vi "Programas.vi"(8 "error in (no error)":errorcluster) -> (0 "error out":errorcluster, 3 "Message":string)   [LabVIEW 2014]
uses:
  controls/Programas/UI Entrenamiento.ctl
  controls/Programas/UI Metabolico.ctl
  controls/Programas/UI Activacion.ctl
  controls/Programas/UI Avatar.ctl
panel:
  out "date/time string":string
  in  "Help":bool
  in  "Reset":bool
  in  "Back":bool
  in  "Avatar":T1 caption="Date Time"
  in  "Activacion":T2
  in  "Metabolico":T3
  in  "Entrenamiento":T4
  # "Elija un Programa"
  # "Presentación"
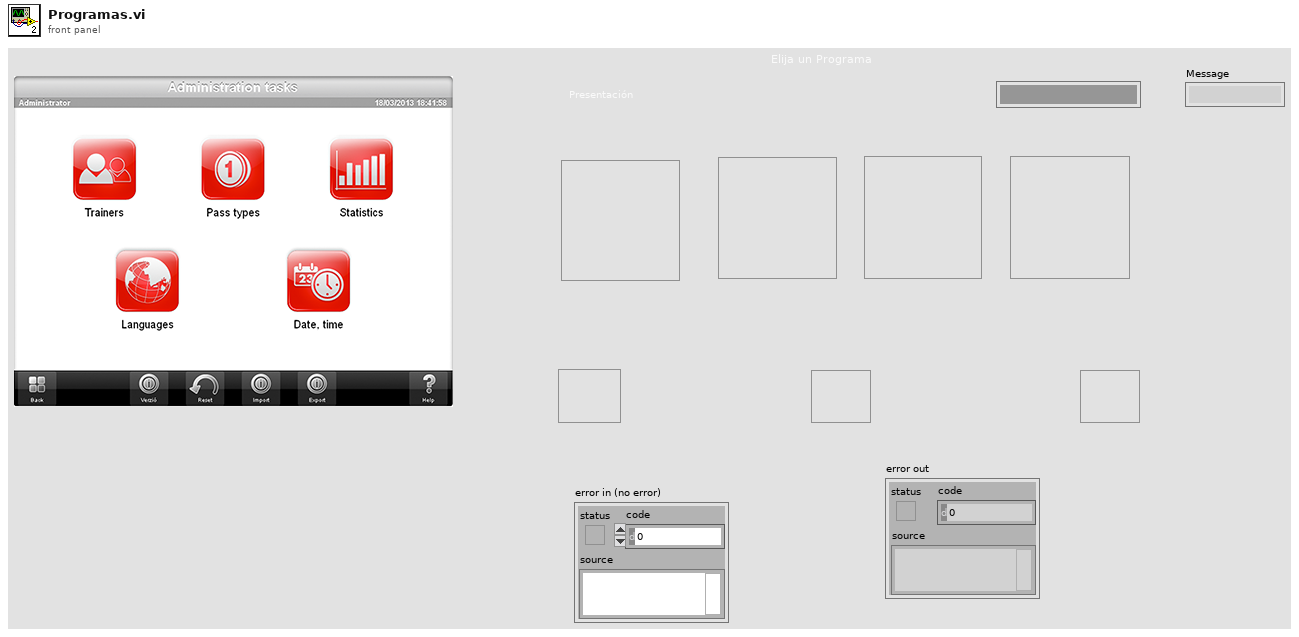
[diagram p1: front panel]
types:
  T1 = typedef "UI Avatar.ctl" = bool
  T2 = typedef "UI Activacion.ctl" = bool
  T3 = typedef "UI Metabolico.ctl" = bool
  T4 = typedef "UI Entrenamiento.ctl" = bool
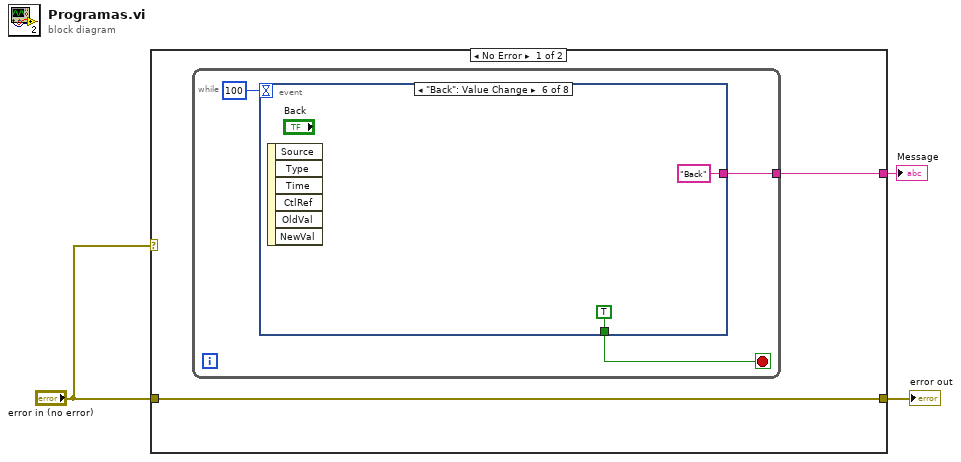
[diagram p0: block diagram]
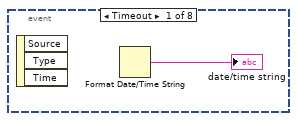
[diagram p2: hidden frame]
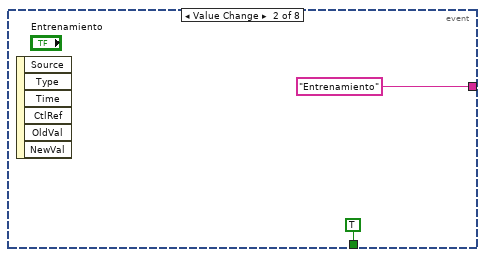
[diagram p3: hidden frame]
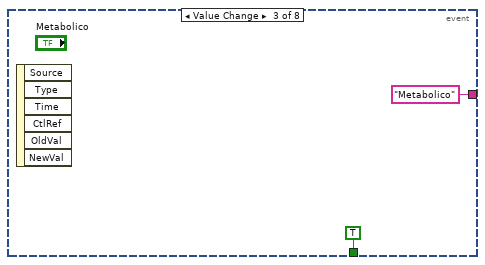
[diagram p4: hidden frame]
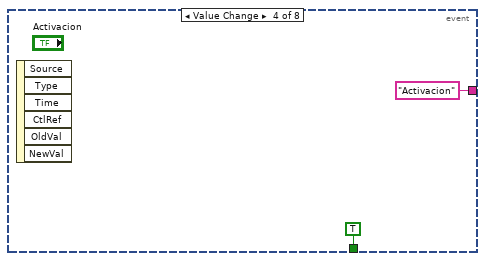
[diagram p5: hidden frame]
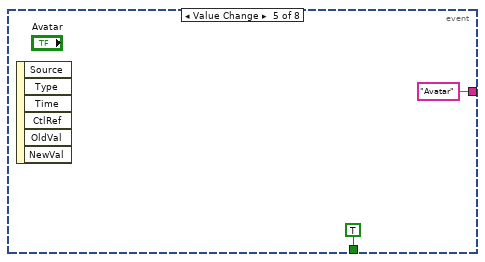
[diagram p6: hidden frame]
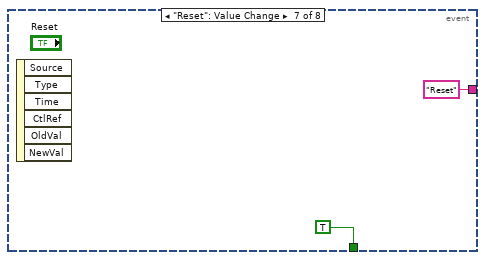
[diagram p7: hidden frame]
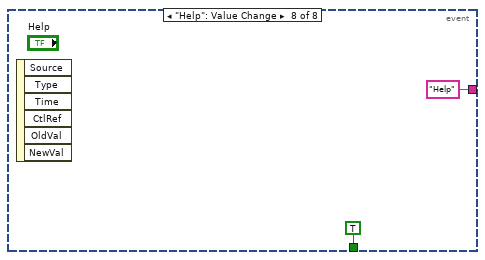
[diagram p8: hidden frame]
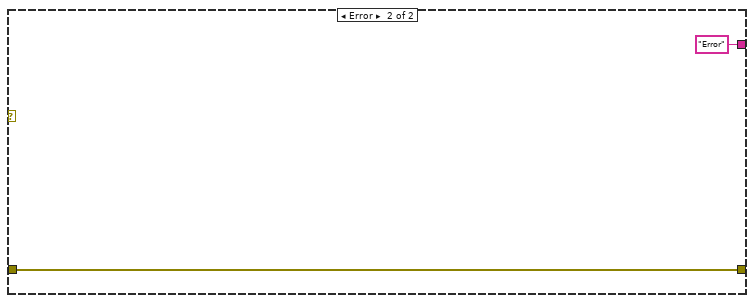
[diagram p9: hidden frame]
diagram:
  n1 = case shown="No Error" "error in (no error)" {
    tunnel: "error in (no error)" -> [w5 w25]
    tunnel: [w5 w25] -> w2
    tunnel: [w4 "Error" ("Message")] -> w1
    frame No Error {
      n2 = while {
        tunnel: [w6] -> w4
        stop <- w8 stop-if-true
        n3 = event shown="[5] \"Back\": Value Change" {
          selector: _ -> [_ _ _ _ _ _ _ _]
          dyn-events: _ -> [_ _ _ _ _ _ _ _]
          timeout: 100 -> [_ _ _ _ _ _ _ _]
          tunnel: [_ TRUE TRUE TRUE TRUE TRUE TRUE TRUE] -> w8
          tunnel: [_ "Entrenamiento" ("Message") "Metabolico" ("Message") "Activacion" ("Message") "Avatar" ("Message") "Back" ("Message") "Reset" ("Message") "Help" ("Message")] -> w6
          event Timeout {
            n4 = event-data() -> ()  [unwired: 1 in, 3 out]
            n5 = Format Date/Time String() -> (date/time string=→"date/time string":string)  [unwired: 3 in]
          }
          event Value Change {
            n6 = event-data() -> ()  [unwired: 1 in, 6 out]
          }
          event Value Change {
            n7 = event-data() -> ()  [unwired: 1 in, 6 out]
          }
          event Value Change {
            n8 = event-data() -> ()  [unwired: 1 in, 6 out]
          }
          event Value Change {
            n9 = event-data() -> ()  [unwired: 1 in, 6 out]
          }
          event "Back": Value Change {
            n10 = event-data() -> ()  [unwired: 1 in, 6 out]
          }
          event "Reset": Value Change {
            n11 = event-data() -> ()  [unwired: 1 in, 6 out]
          }
          event "Help": Value Change {
            n12 = event-data() -> ()  [unwired: 1 in, 6 out]
          }
        }
      }
    }
    frame Error {
    }
  }
  "error out" <- w2
  "Message" <- w1
